vi "Num2BoolArray.vi"(1 "Real 2D Array":u32[][](array[numeric])) -> (0 "BooleanArray":bool[][](array[boolean]))   [LabVIEW 2014]
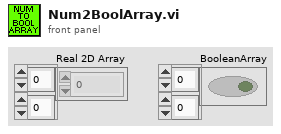
[diagram p1: front panel]
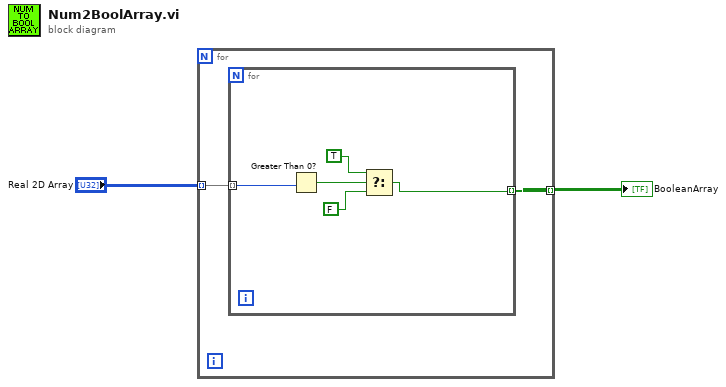
[diagram p0: block diagram]
diagram:
  n1 = for {
    tunnel: "Real 2D Array" -> [w4] mode=indexing
    tunnel: [w3] -> w2 mode=indexing
    n2 = for {
      tunnel: w4 -> [w9] mode=indexing
      tunnel: [w6] -> w3 mode=indexing
      n3 = Greater Than 0?(x=w9) -> (x > 0?=w8:bool)
      n4 = Select(t=TRUE, s=w8, f=FALSE) -> (s? t:f=w6:bool)
    }
  }
  "BooleanArray" <- w2
